vi "AddToDeviceEnqueuerList.vi"(8 "error in (no error)":errorcluster, 9 "Label":string, 10 "DeviceEnqueuer":refnum<class "Message Enqueuer.lvclass">, 11 "Microscope in":refnum<class "Microscope.lvclass">) -> (0 "error out":errorcluster, 1 "value unchanged?":bool, 2 "key already included?":bool, 3 "Microscope out":refnum<class "Microscope.lvclass">)   [LabVIEW 2020, in "Microscope.lvlib" / "Microscope.lvclass"]
uses:
  Microscope.lvclass
  <vilib>/ActorFramework/Message Enqueuer/Message Enqueuer.lvclass
  Microscope.lvclass/Microscope.ctl
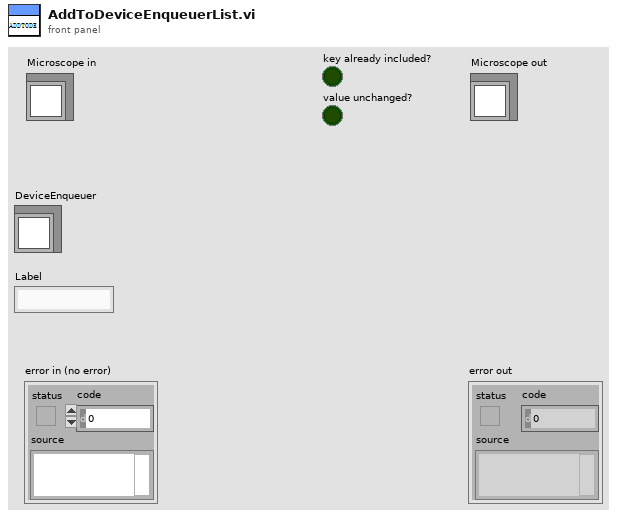
[diagram p1: front panel]
types:
  T1 = map{string, refnum<class "Message Enqueuer.lvclass">}
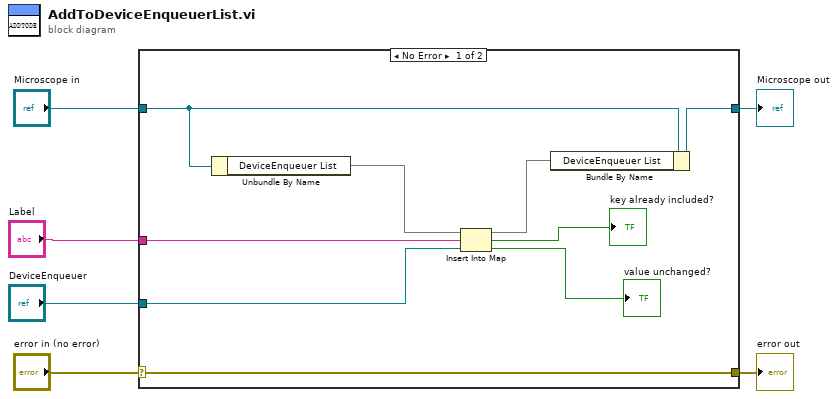
[diagram p0: block diagram]
diagram:
  n1 = case shown="No Error" "error in (no error)" {
    selector: "error in (no error)" -> [w15 w17]
    tunnel: [w15 w17] -> w5
    tunnel: [w10 w16] -> w3
    tunnel: "Microscope in" -> [w14 w16]
    tunnel: "Label" -> [w12 _]
    tunnel: "DeviceEnqueuer" -> [w11 _]
    frame No Error {
      n2 = Unbundle By Name(w14) -> ("DeviceEnqueuer List"=w13:T1)
      n3 = Insert Into Map(map in=w13, key=w12, value=w11) -> (map out=w9:T1, key already included?=→"key already included?":bool, value unchanged?=→"value unchanged?":bool)
      n4 = Bundle By Name(cluster=w14, "DeviceEnqueuer List"=w9) -> (w10:refnum<class "Microscope.lvclass">)
    }
    frame Error {
    }
  }
  "error out" <- w5
  "Microscope out" <- w3
